vi "move-ABS-RAW.vi"(10 "position":dbl, 11 "Device in":refnum<k24>) -> (3 "Device out":refnum<k24>)   [LabVIEW 2014]
uses:
  C:/user-Lab/AndreTec/GITs/andretec/Thorlabs-Vector-Move/kinesisTec/Kinesis/Thorlabs.MotionControl.TCube.DCServoCLI.dll
  kinesisTec/Kinesis/Thorlabs.MotionControl.TCube.DCServoCLI.dll
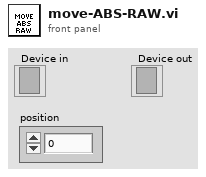
[diagram p1: front panel]
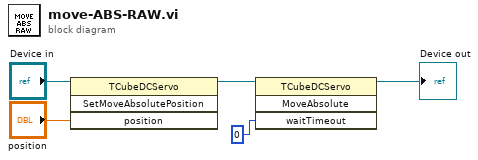
[diagram p0: block diagram]
diagram:
  n1 = invoke class="TCubeDCServo" method="SetMoveAbsolutePosition"(reference="Device in", "position"="position") -> (reference out=w3:refnum<k24>)  [unwired: 2 in, 3 out]
  n2 = invoke class="TCubeDCServo" method="MoveAbsolute"(reference=w3, "waitTimeout"=0) -> (reference out=→"Device out":refnum<k24>)  [unwired: 2 in, 3 out]
